vi "Change User Pwd.vi"(8 "error in (no error)":errorcluster, 9 "Password":string, 10 "Username":string, 11 "UserPwd DB in":refnum<class "UserPwd DB.lvclass">) -> (0 "error out":errorcluster, 2 "changed":bool, 3 "UserPwd DB out":refnum<class "UserPwd DB.lvclass">)   [LabVIEW 2016, in "UserPwd DB.lvlib" / "UserPwd DB.lvclass"]
uses:
  <userlib>/Common Components/UserPwd DB/UserPwd DB/UserPwd DB.lvclass
  <userlib>/Common Components/UserPwd DB/UserPwd DB/UserPwd DB.lvclass/UserPwd DB.ctl
  <userlib>/Common Components/UserPwd DB/UserPwd DB/Data saved.ctl
  <userlib>/Common Components/UserPwd DB/UserPwd DB/Access Level.ctl
  <vilib>/addons/_JKI.lib/Serialization/JSON/JKI JSON Serialization.lvlib
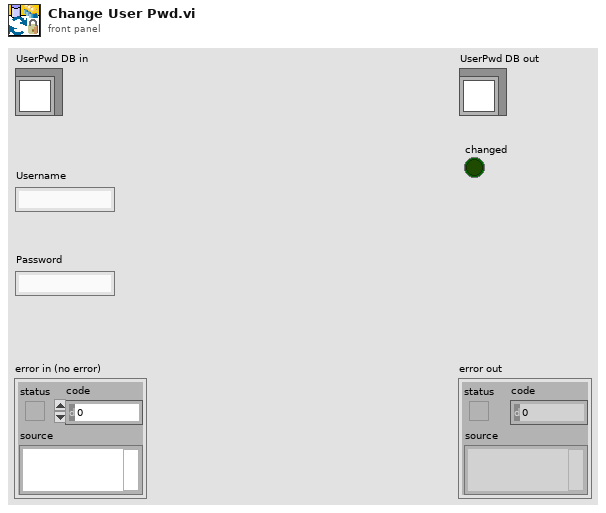
[diagram p1: front panel]
types:
  T1 = typedef "UserPwd DB.lvlib/UserPwd DB.lvclass/Data saved.ctl" = cluster{"Encrypted Password":string, "Access":T2, "Permission":u32}
  T2 = typedef "UserPwd DB.lvlib/UserPwd DB.lvclass/Access Level.ctl" = enum16{"Admin", "User lv1", "User lv2", "User lv3", "User lv4", "User lv5", "User lv6", "User lv7", "User lv8", "User lv9", "Guest"}
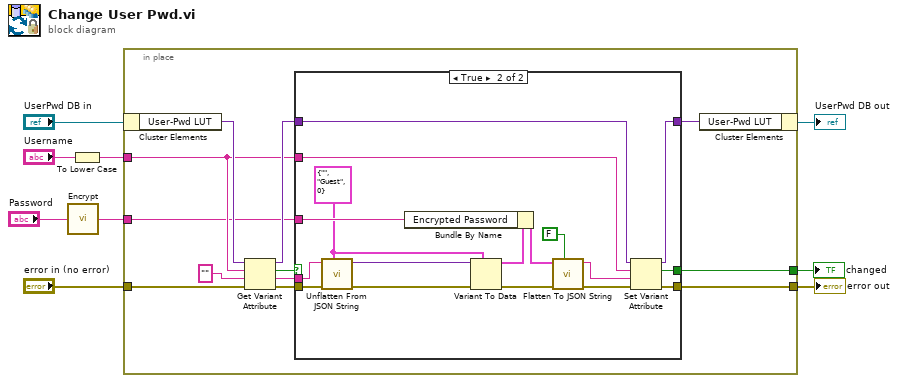
[diagram p0: block diagram]
diagram:
  n1 = call <userlib>:"Encrypt.vi"("String"="Password") -> ("Encrypted String"=w2:string)
  n2 = To Lower Case(string="Username") -> (all lower case string=w1:string)
  n3 = in-place {
    in-place-border: w1 -> [w17]
    in-place-border: "error in (no error)" -> [w19]
    in-place-border: [w12] -> w5
    in-place-border: [w14] -> w4
    in-place-border: w2 -> [w15]
    n4 = in-place-cluster #1("UserPwd DB in") -> ("User-Pwd LUT"=w21:variant)
    n5 = Get Variant Attribute(Variant=w21, name=w17, default value (empty Variant)="" ("Password"), error in=w19) -> (duplicate Variant=w20:variant, found=w11:bool, value=w16:string, error out=w13:errorcluster)
    n6 = case shown="True" w11 {
      tunnel: w20 -> [w23 w40]
      tunnel: [w23 w39] -> w18
      tunnel: w17 -> [_ w38]
      tunnel: w16 -> [_ w30]
      tunnel: w15 -> [_ w37]
      tunnel: [_ w36] -> w14
      tunnel: w13 -> [w22 w35]
      tunnel: [w22 w34] -> w12
      frame False {
      }
      frame True {
        w29 = T1 {"Encrypted Password"="", "Access"=enum."Guest", "Permission"=0} ("Data")
        n7 = call <vilib>:"Unflatten From JSON String.vi"("Type and Defaults"=w29, "error in (no error)"=w35, "JSON String"=w30) -> ("error out"=w33:errorcluster, "Variant"=w28:variant)  [unwired: 7 in]
        n8 = Variant To Data(error in=w33, type=w29, Variant=w28) -> (data=w27:T1, error out=w32:errorcluster)
        n9 = Bundle By Name(cluster=w27, "Encrypted Password"=w37) -> (w26:T1)
        n10 = call <vilib>:"Flatten To JSON String.vi"("Multiline (T)"=FALSE, "error in (no error)"=w32, "Variant"=w26) -> ("error out"=w31:errorcluster, "JSON String"=w25:string)  [unwired: 7 in]
        n11 = Set Variant Attribute(Variant=w40, name=w38, value=w25, error in=w31) -> (Variant out=w39:variant, replaced=w36:bool, error out=w34:errorcluster)
      }
    }
    n12 = in-place-cluster #1("User-Pwd LUT"=w18) -> (→"UserPwd DB out":refnum<class "UserPwd DB.lvclass">)
  }
  "error out" <- w5
  "changed" <- w4
